vi "Fit.vi"(8 "error in (no error)":errorcluster caption="entrée d'erreur (pas d'erreur)", 10 "y":string[][](array[string]), 11 "LabelEncoder.lvclass":refnum<class "LabelEncoder.lvclass">) -> (0 "error out":errorcluster caption="sortie d'erreur", 2 "String Data":string, 3 "LabelEncoder.lvclass":refnum<class "LabelEncoder.lvclass">)   [LabVIEW 2020, in "LabelEncoder.lvclass"]
doc: "Fit label encoder : \n\nReturns : \n\n- String : OK"
uses:
  LabelEncoder.lvclass
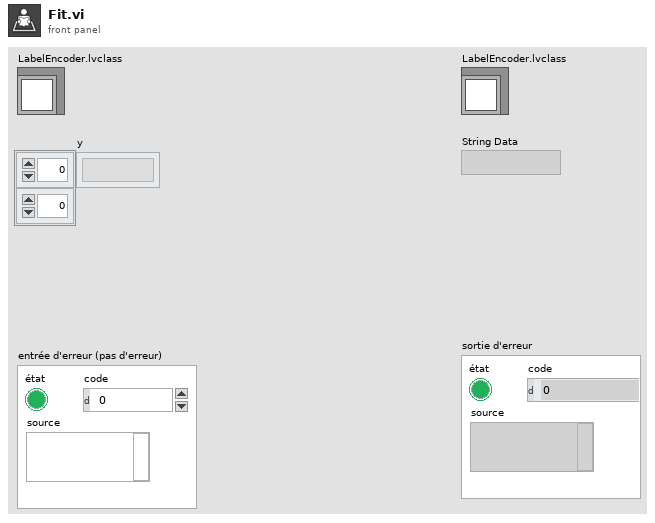
[diagram p1: front panel]
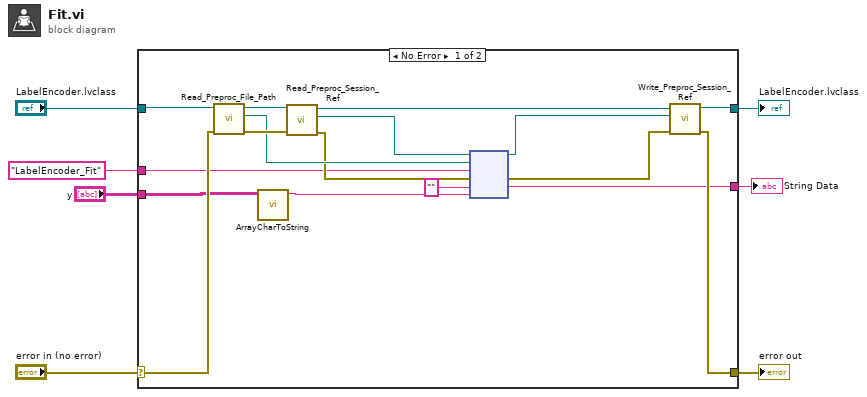
[diagram p0: block diagram]
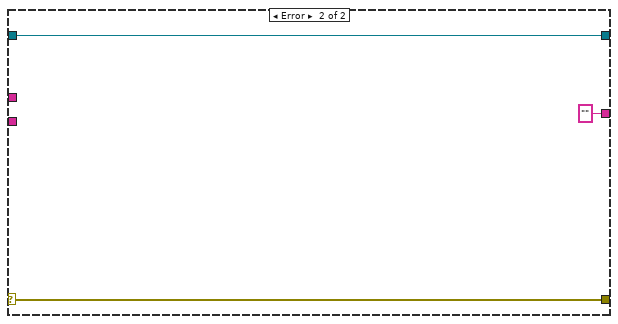
[diagram p2: hidden frame]
diagram:
  n1 = case shown="No Error" "error in (no error)" {
    selector: "error in (no error)" -> [w14 w27]
    tunnel: [w13 w27] -> w6
    tunnel: [w15 w26] -> w4
    tunnel: "LabelEncoder.lvclass" -> [w12 w26]
    tunnel: "LabelEncoder_Fit" ("Fonction") -> [w11 _]
    tunnel: [w10 ""] -> w2
    tunnel: "y" -> [w9 _]
    frame No Error {
      n2 = call-dynamic "Read_Preproc_File_Path.vi"("error in (no error)"=w14, "Python in"=w12) -> ("error out"=w23:errorcluster, "File_Path"=w20:path, "Python out"=w24:refnum<class "LabelEncoder.lvclass">)  [unwired: 7 in]
      n3 = call "ArrayCharToString.vi"("TAB"=w9) -> ("Instruction"=w8:string)  [unwired: 10 in]
      n4 = call-dynamic "Read_Preproc_Session_Ref.vi"("error in (no error)"=w23, "Python in"=w24) -> ("error out"=w19:errorcluster, "Session_ref"=w21:refnum<k35>, "Python out"=w22:refnum<class "LabelEncoder.lvclass">)  [unwired: 7 in]
      n5 = node(w21, w20, w11, w19, "", w8) -> (w17:refnum<k35>, w18:errorcluster, w10:string)  [unwired: 1 in, 2 out]
      n6 = call-dynamic "Write_Preproc_Session_Ref.vi"("error in (no error)"=w18, "Session_ref"=w17, "Python in"=w22) -> ("error out"=w13:errorcluster, "Python out"=w15:refnum<class "LabelEncoder.lvclass">)  [unwired: 7 in]
    }
    frame Error {
    }
  }
  "error out" <- w6
  "LabelEncoder.lvclass" <- w4
  "String Data" <- w2
